vi "Caveat 1 Fix.vi"() -> ()   [LabVIEW 2025]
uses:
  Caveat 1 - States.ctl
panel:
  out "Option 2 Selected?":bool
  out "Option 1 Selected?":bool
  out "Loop Iterations":i32
  in  "Reset Error":bool
  out "Error Msg":errorcluster
  in  "Option 2 Controls":T1
  in  "Option 1 Controls":T2
  in  "Option 1":bool
  in  "Option 2":bool
  # "Caveat 1: Avoid UI Propert Nodes (Error 1055)"
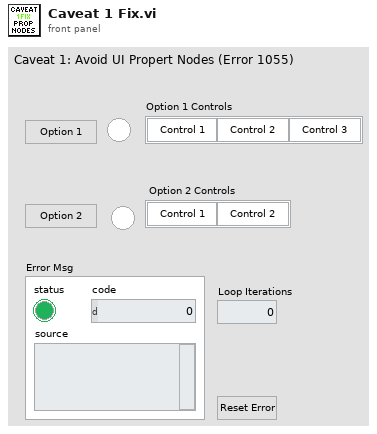
[diagram p1: front panel]
types:
  T1 = cluster{"Option 2, ctrl 1":bool, "Option 2, ctrl 2":bool}
  T2 = cluster{"Option 1, ctrl 1":bool, "Option 1, ctrl 2":bool, "Option 1, ctrl 3":bool}
  T3 = typedef "Caveat 1 - States.ctl" = enum16{"Init", "Poll UI", "Option 1 Selected", "Option 2 Selected", "Error", "Reset Error"}
  T4 = enum8{"Enabled", "Disabled", "Disabled and Grayed Out"}
  T5 = enum16{"Option 1 Btn", "Option 2 Btn", "Option 1 Ctrls", "Option 2 Ctrls"}
  T6 = enum16{"Option 1 Btn", "Option 2 Btn", "Option 1 Ctrls", "Option 2 Ctrls"}[]
  T7 = enum8{"Enabled", "Disabled", "Disabled and Grayed Out"}[]
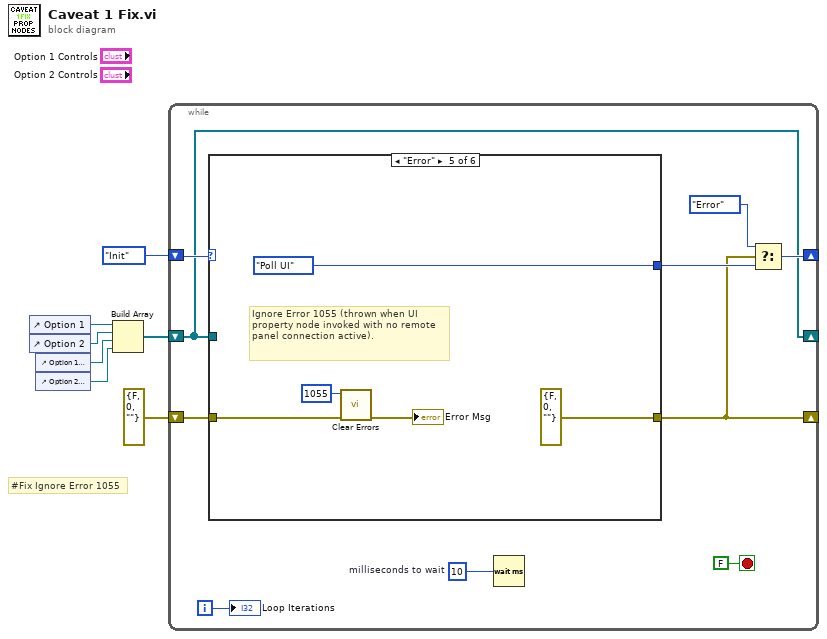
[diagram p0: block diagram]
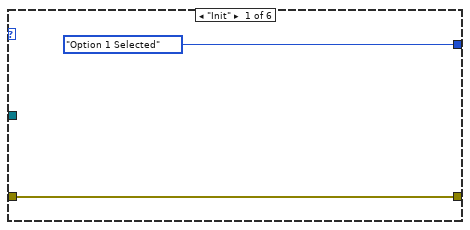
[diagram p2: hidden frame]
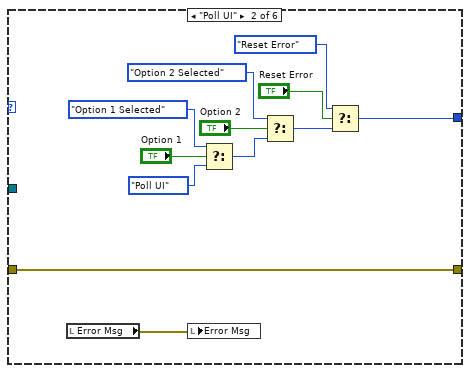
[diagram p3: hidden frame]
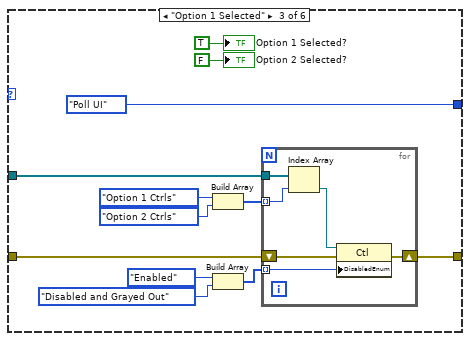
[diagram p4: hidden frame]
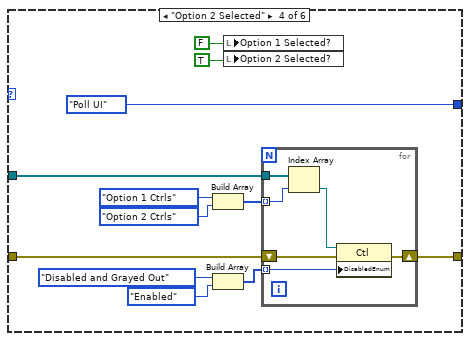
[diagram p5: hidden frame]
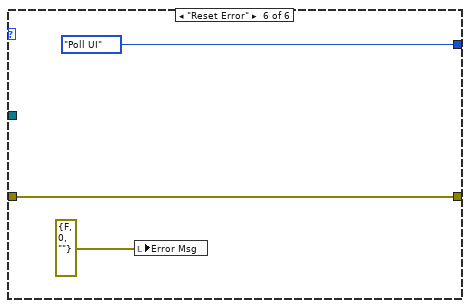
[diagram p6: hidden frame]
diagram:
  # "#Fix Ignore Error 1055"
  n1 = control-ref of="Option 1"() -> (w6:refnum<vi>)
  n2 = control-ref of="Option 2"() -> (w5:refnum<vi>)
  n3 = control-ref of="Option 1 Controls"() -> (w3:refnum<vi>)
  n4 = control-ref of="Option 2 Controls"() -> (w2:refnum<vi>)
  n5 = Build Array(w6, w5, w3, w2) -> (w4:refnum<vi>[])
  n6 = while {
    shift-right: [w12] -> _
    shift-left: Caveat_1_-_States."Init" -> [w15]
    shift-right: [w11] -> _
    shift-left: errorcluster {"status"=FALSE, "code"=0, "source"=""} ("error IO") -> [w10]
    shift-right: [w8] -> _
    shift-left: w4 -> [w8]
    i -> [w9]
    stop <- FALSE stop-if-true
    w16 = u32 10  # milliseconds to wait
    n7 = case shown="\"Error\"" w15 {
      tunnel: w8 -> [_ _ w34 w52 _ _]
      tunnel: [Caveat_1_-_States."Option 1 Selected" w20 Caveat_1_-_States."Poll UI" Caveat_1_-_States."Poll UI" Caveat_1_-_States."Poll UI" Caveat_1_-_States."Poll UI"] -> w13
      tunnel: [w18 w24 w40 w58 errorcluster {"status"=FALSE, "code"=0, "source"=""} ("error IO") w74] -> w11
      tunnel: w10 -> [w18 w24 w35 w53 w70 w74]
      frame "Init" {
      }
      frame "Poll UI" {
        n8 = local read "Error Msg"() -> (w25:errorcluster)
        n9 = local write "Error Msg"(w25) -> ()
        n10 = Select(t=Caveat_1_-_States."Option 1 Selected", s="Option 1", f=Caveat_1_-_States."Poll UI") -> (s? t:f=w29:T3)
        n11 = Select(t=Caveat_1_-_States."Option 2 Selected", s="Option 2", f=w29) -> (s? t:f=w23:T3)
        n12 = Select(t=Caveat_1_-_States."Reset Error", s="Reset Error", f=w23) -> (s? t:f=w20:T3)
      }
      frame "Option 1 Selected" {
        n13 = Build Array(T5."Option 1 Ctrls", T5."Option 2 Ctrls") -> (w43:T6)
        n14 = Build Array(T4."Enabled" ("Disabled"), T4."Disabled and Grayed Out" ("Disabled")) -> (w36:T7)
        n15 = for {
          tunnel: w43 -> [w48] mode=indexing
          tunnel: w34 -> [w49]
          tunnel: w36 -> [w46] mode=indexing
          shift-right: [w45] -> w40
          shift-left: w35 -> [w44]
          n16 = Index Array(array=w49, index=w48) -> (element=w47:refnum<vi>)
          n17 = property class="Ctl"(reference=w47, error in=w44, "DisabledEnum"=w46) -> (error out=w45:errorcluster)  [unwired: 1 out]
        }
        "Option 1 Selected?" <- TRUE
        "Option 2 Selected?" <- FALSE
      }
      frame "Option 2 Selected" {
        n18 = Build Array(T5."Option 1 Ctrls", T5."Option 2 Ctrls") -> (w61:T6)
        n19 = Build Array(T4."Disabled and Grayed Out" ("Disabled"), T4."Enabled" ("Disabled")) -> (w54:T7)
        n20 = local write "Option 1 Selected?"(FALSE) -> ()
        n21 = local write "Option 2 Selected?"(TRUE) -> ()
        n22 = for {
          tunnel: w61 -> [w66] mode=indexing
          tunnel: w52 -> [w67]
          tunnel: w54 -> [w64] mode=indexing
          shift-right: [w63] -> w58
          shift-left: w53 -> [w62]
          n23 = Index Array(array=w67, index=w66) -> (element=w65:refnum<vi>)
          n24 = property class="Ctl"(reference=w65, error in=w62, "DisabledEnum"=w64) -> (error out=w63:errorcluster)  [unwired: 1 out]
        }
      }
      frame "Error" {
        # "Ignore Error 1055 (thrown when UI property node invoked with no remote panel connection active)."
        n25 = call <vilib>:"Clear Errors.vi"("error in (no error)"=w70, "specific error code to clear (0: all)"=1055) -> ("error out"=→"Error Msg":errorcluster)  [unwired: 4 in, 1 out]
      }
      frame "Reset Error" {
        n26 = local write "Error Msg"(errorcluster {"status"=FALSE, "code"=0, "source"=""} ("error IO")) -> ()
      }
    }
    n27 = Wait (ms)(milliseconds to wait=w16) -> ()  [unwired: 1 out]
    n28 = Select(t=Caveat_1_-_States."Error", s=w11, f=w13) -> (s? t:f=w12:T3)
    "Loop Iterations" <- w9
  }
